vi "Parse Task Details.vi"(0 "Task details XML":string, 5 "error in (no error)":errorcluster) -> (8 "command":string, 10 "arguments":string, 11 "EWI href":string, 12 "advsettings":string, 14 "Task type":string, 16 "resultURL":string, 17 "remotescript href":string, 19 "error out":errorcluster)   [LabVIEW 2012]
uses:
  <vilib>/xml/Load XML String.vi
  <vilib>/xml/Close Reference(Node).vi
  <vilib>/xml/NI_XML.lvlib
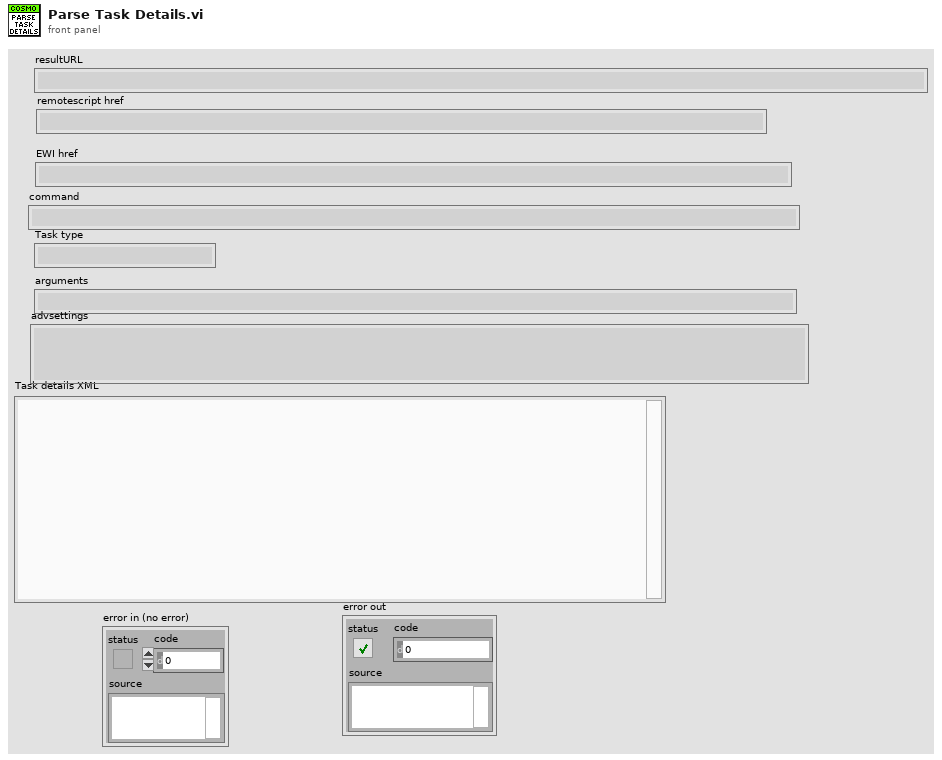
[diagram p1: front panel]
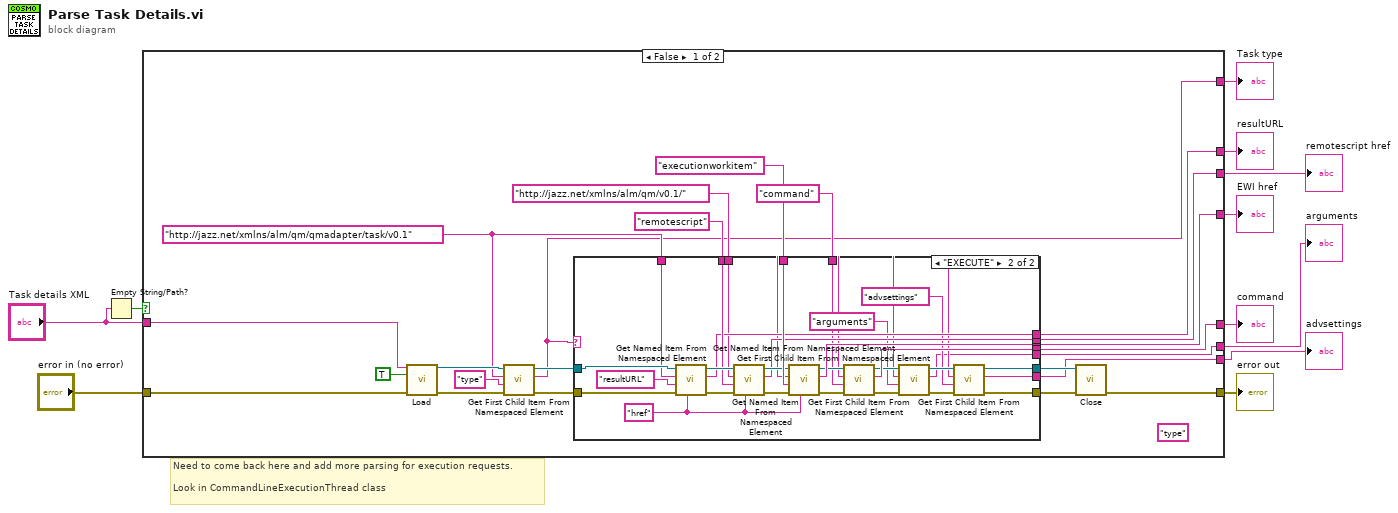
[diagram p0: block diagram]
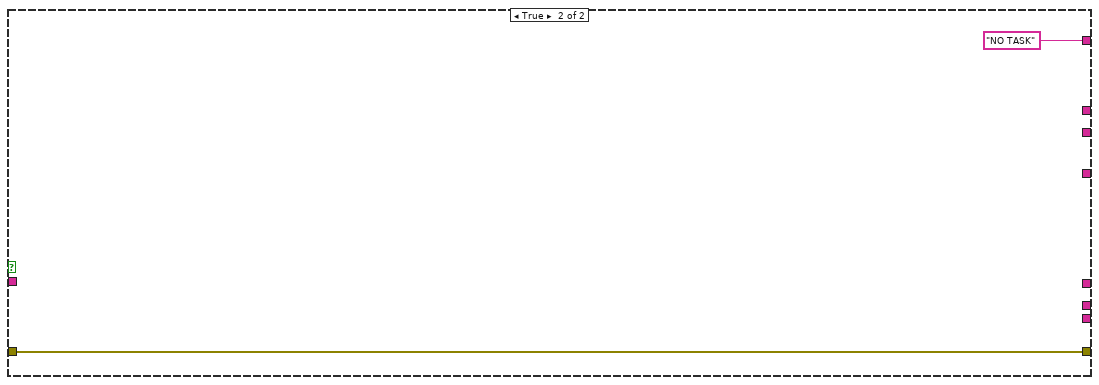
[diagram p3: hidden frame]
diagram:
  # "Need to come back here and add more parsing for execution requests.\n\nLook in CommandLineExecutionThread class"
  n1 = Empty String/Path?(string/path="Task details XML") -> (empty?=w8:bool)
  n2 = case shown="False" w8 {
    tunnel: "Task details XML" -> [w34 _]
    tunnel: [w12 "NO TASK" ("Value")] -> w11
    tunnel: "error in (no error)" -> [w32 w67]
    tunnel: [w29 w67] -> w9
    tunnel: [w28 _] -> w6
    tunnel: [w27 _] -> w5
    tunnel: [w26 _] -> w4
    tunnel: [w18 _] -> w3
    tunnel: [w14 _] -> w1
    tunnel: [w13 _] -> w2
    frame False {
      w15 = "http://jazz.net/xmlns/alm/qm/qmadapter/task/v0.1"
      (unwired) "type" ("Local Name")
      n3 = call-poly <vilib>:"Load.vi"("XML string"=w34, "process namespaces (False)"=TRUE, "error in (no error)"=w32) -> ("DOM document out"=w24:refnum<k20>, "error out"=w25:errorcluster)  [unwired: 10 in, 1 out]
      n4 = call "Get First Child Item From Namespaced Element.vi"("error in (no error)"=w25, "Local Name"="type", "Namespace URI"=w15, "DOM document in"=w24) -> ("error out"=w21:errorcluster, "Value"=w12:string, "DOM document out"=w23:refnum<k20>)  [unwired: 5 in]
      n5 = case shown="\"EXECUTE\"" w12 {
        tunnel: "remotescript" ("Local Name") -> [_ w63]
        tunnel: "executionworkitem" ("Local Name") -> [_ w61]
        tunnel: [_ w58] -> w28
        tunnel: [_ w57] -> w27
        tunnel: [_ w56] -> w26
        tunnel: w23 -> [w36 w55]
        tunnel: w21 -> [w35 w54]
        tunnel: "http://jazz.net/xmlns/alm/qm/v0.1/" ("Local Name") -> [_ w53]
        tunnel: "command" ("Local Name") -> [_ w50]
        tunnel: [_ w49] -> w18
        tunnel: [w36 w43] -> w17
        tunnel: [w35 w42] -> w16
        tunnel: w15 -> [_ w40]
        tunnel: [_ w39] -> w14
        tunnel: [_ w38] -> w13
        frame Default {
        }
        frame "EXECUTE" {
          w37 = "href" ("Tag")
          n6 = call "Get Named Item From Namespaced Element.vi"("Tag"=w37, "error in (no error)"=w54, "Local Name"="resultURL", "Namespace URI"=w40, "DOM document in"=w55) -> ("error out"=w62:errorcluster, "Value"=w56:string, "DOM document out"=w64:refnum<k20>)  [unwired: 4 in]
          n7 = call "Get Named Item From Namespaced Element.vi"("Tag"=w37, "error in (no error)"=w62, "Local Name"=w63, "Namespace URI"=w53, "DOM document in"=w64) -> ("error out"=w60:errorcluster, "Value"=w57:string, "DOM document out"=w59:refnum<k20>)  [unwired: 4 in]
          n8 = call "Get Named Item From Namespaced Element.vi"("Tag"=w37, "error in (no error)"=w60, "Local Name"=w61, "Namespace URI"=w53, "DOM document in"=w59) -> ("error out"=w51:errorcluster, "Value"=w58:string, "DOM document out"=w52:refnum<k20>)  [unwired: 4 in]
          n9 = call "Get First Child Item From Namespaced Element.vi"("error in (no error)"=w51, "Local Name"=w50, "Namespace URI"=w40, "DOM document in"=w52) -> ("error out"=w47:errorcluster, "Value"=w49:string, "DOM document out"=w48:refnum<k20>)  [unwired: 5 in]
          n10 = call "Get First Child Item From Namespaced Element.vi"("error in (no error)"=w47, "Local Name"="arguments", "Namespace URI"=w40, "DOM document in"=w48) -> ("error out"=w44:errorcluster, "Value"=w38:string, "DOM document out"=w45:refnum<k20>)  [unwired: 5 in]
          n11 = call "Get First Child Item From Namespaced Element.vi"("error in (no error)"=w44, "Local Name"="advsettings", "Namespace URI"=w40, "DOM document in"=w45) -> ("error out"=w42:errorcluster, "Value"=w39:string, "DOM document out"=w43:refnum<k20>)  [unwired: 5 in]
        }
      }
      n12 = call-poly <vilib>:"Close.vi"("error in (no error)"=w16, "node"=w17) -> ("error out"=w29:errorcluster)  [unwired: 7 in]
    }
    frame True {
    }
  }
  "Task type" <- w11
  "error out" <- w9
  "resultURL" <- w4
  "remotescript href" <- w5
  "EWI href" <- w6
  "command" <- w3
  "arguments" <- w2
  "advsettings" <- w1
